vi "Equal - RM,RM.vi"(1 "Real Matrix B":T1, 2 "Real Matrix A":T1) -> (0 "A = B?":bool)   [LabVIEW 2017, in "NI_Matrix.lvlib"]
doc: "Returns TRUE if <B>x</B> is equal to <B>y</B>. Otherwise, this function returns FALSE."
uses:
  <vilib>/Analysis/Matrix/NI_Matrix.lvlib
  <vilib>/Analysis/Matrix/Datatypes/RealMatrix.ctl
  <vilib>/Analysis/Matrix/Numeric/Conversions/Matrix To Array - RM.vi
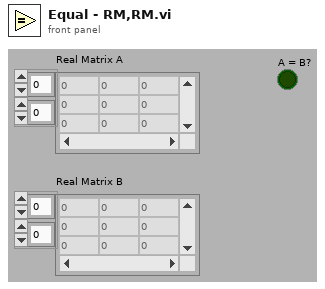
[diagram p1: front panel]
types:
  T1 = typedef "NI_Matrix.lvlib/RealMatrix.ctl" = dbl[][]
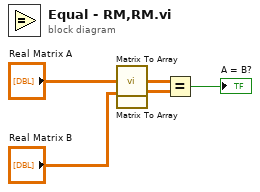
[diagram p0: block diagram]
diagram:
  n1 = call-poly <vilib>:"Matrix To Array.vi"("Real Matrix"="Real Matrix A") -> ("Real 2D Array"=w3:dbl[][])
  n2 = call-poly <vilib>:"Matrix To Array.vi"("Real Matrix"="Real Matrix B") -> ("Real 2D Array"=w2:dbl[][])
  n3 = Equal?(x=w3, y=w2) -> (x = y?=→"A = B?":bool)
